vi "Unpack Digital Command.vi"(8 "error in (no error)":errorcluster, 9 "Data":variant, 10 "Type":string, 11 "Module in":refnum<class "Module.lvclass">) -> (0 "error out":errorcluster, 1 "Remote":bool, 2 "CmdDigitalMultiple":T2, 3 "Module out":refnum<class "Module.lvclass">, 5 "TcpPayload":T1)   [LabVIEW 2023, in "Volatus.lvlib" / "Module.lvclass"]
uses:
  Module.lvclass
  messages/CmdDigitalMultiple/Data.ctl
  messages/CmdDigital/Data.ctl
  lv-vecto/Vecto/proto/TcpPayload/Data.ctl
  messages/CmdDigitalMultiple/Class/Msg.lvclass
  C:/dev/volatus/mts-volatus-super/libs/lv-protoc/LV-Proto/Message/Message.lvclass
  messages/CmdDigitalMultiple/Class/Msg.lvclass/Msg.ctl
  messages/CmdDigital/CmdDigital.lvlib
  messages/CmdDigitalMultiple/CmdDigitalMultiple.lvlib
  lv-vecto/Vecto/proto/TcpPayload/TcpPayload.lvlib
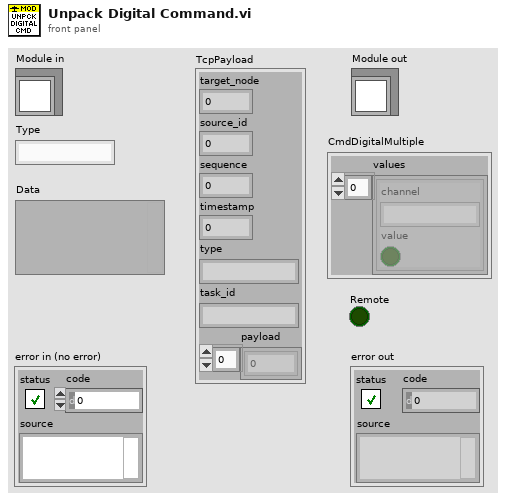
[diagram p1: front panel]
types:
  T1 = typedef "TcpPayload.lvlib/Data.ctl" = cluster{"target_node":u32, "source_id":u32, "sequence":u32, "timestamp":i64, "type":string, "task_id":string, "payload":u8[]}
  T2 = typedef "CmdDigitalMultiple.lvlib/Data.ctl" = cluster{"values":T3[]}
  T3 = typedef "CmdDigital.lvlib/Data.ctl" = cluster{"channel":string, "value":bool}
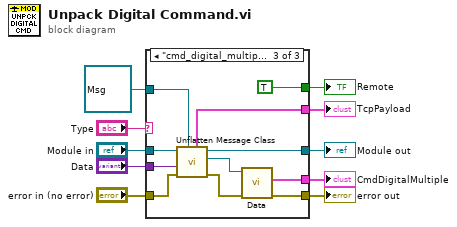
[diagram p0: block diagram]
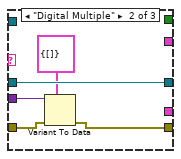
[diagram p3: hidden frame]
diagram:
  n1 = case shown="\"cmd_digital_multiple\"" "Type" {
    tunnel: "Data" -> [_ w16 w25]
    tunnel: "error in (no error)" -> [w11 w15 w24]
    tunnel: "Module in" -> [w12 w17 w28]
    tunnel: [w12 w17 w27] -> w6
    tunnel: [_ _ TRUE] -> w5
    tunnel: [w11 w14 w19] -> w4
    tunnel: refnum<class "Msg.lvclass"> refnum ("CmdDigitalMultiple.lvlib:Msg.lvclass") -> [_ _ w23]
    tunnel: [_ _ w22] -> w2
    tunnel: [_ _ w18] -> w1
    frame Default {
    }
    frame "Digital Multiple" {
      n2 = Variant To Data(error in=w15, type=T2 {"values"=[]} ("Data"), Variant=w16) -> (error out=w14:errorcluster)  [unwired: 1 out]
    }
    frame "cmd_digital_multiple" {
      n3 = call "Unflatten Message Class.vi"("Message Type"=w23, "error in (no error)"=w24, "Data"=w25, "Module in"=w28) -> ("error out"=w20:errorcluster, "Message"=w21:refnum<class "Msg.lvclass">, "Module out"=w27:refnum<class "Module.lvclass">, "TcpPayload"=w22:T1)  [unwired: 4 in]
      n4 = call "Data.vi"("error in (no error)"=w20, "PB Msg Template in"=w21) -> ("error out"=w19:errorcluster, "Data"=w18:T2)  [unwired: 7 in, 1 out]
    }
  }
  "error out" <- w4
  "Module out" <- w6
  "CmdDigitalMultiple" <- w1
  "Remote" <- w5
  "TcpPayload" <- w2
